vi "Teleop Climb Control.vi"(9 "D-Pad":T1, 10 "Button Cluster":T2, 11 "Axes":T3) -> ()   [LabVIEW 2017]
uses:
  Common Code/Gamepads/Axes Cluster.ctl
  Common Code/Gamepads/Button Cluster.ctl
  Common Code/Gamepads/D-Pad.ctl
  Common Code/Climb Command Cluster.ctl
  Common Code/Utilities/Change Detect.vi
  Common Code/Utilities/Change Detect Boolean.vi
  Robot Global Data.vi
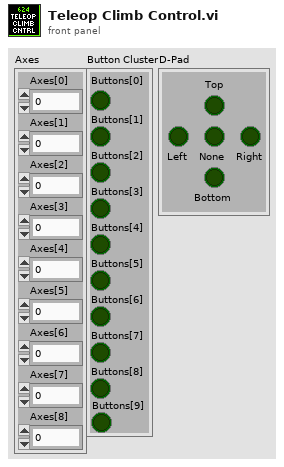
[diagram p1: front panel]
types:
  T1 = typedef "D-Pad.ctl" = cluster{"Top":bool, "Bottom":bool, "None":bool, "Right":bool, "Left":bool}
  T2 = typedef "Button Cluster.ctl" = cluster{"Buttons[0]":bool, "Buttons[1]":bool, "Buttons[2]":bool, "Buttons[3]":bool, "Buttons[4]":bool, "Buttons[5]":bool, "Buttons[6]":bool, "Buttons[7]":bool, "Buttons[8]":bool, "Buttons[9]":bool}
  T3 = typedef "Axes Cluster.ctl" = cluster{"Axes[0]":dbl, "Axes[1]":dbl, "Axes[2]":dbl, "Axes[3]":dbl, "Axes[4]":dbl, "Axes[5]":dbl, "Axes[6]":dbl, "Axes[7]":dbl, "Axes[8]":dbl}
  T4 = typedef "Climb Command Cluster.ctl" = cluster{"Climb":bool, "Button Pressed":bool}
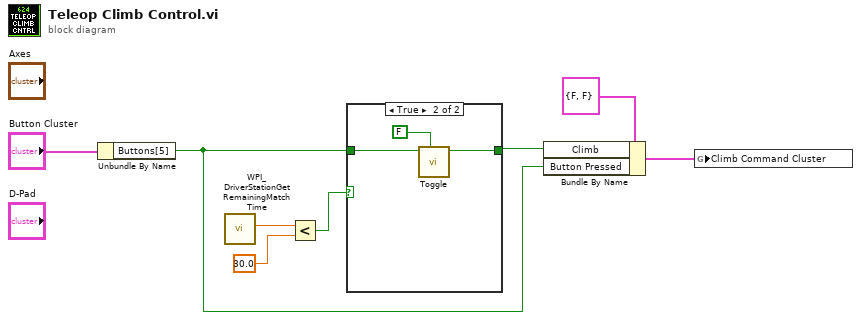
[diagram p0: block diagram]
diagram:
  n1 = Unbundle By Name("Button Cluster") -> ("Buttons[5]"=w2:bool)
  n2 = call <vilib>:"WPI_DriverStationGetRemainingMatchTime.vi"() -> ("Match Time(s)"=w1:sgl)  [unwired: 10 in, 1 out]
  n3 = Less?(x=w1, y=sgl 30.0) -> (x < y?=w3:bool)
  n4 = case shown="True" w3 {
    tunnel: [_ w9] -> w4
    tunnel: w2 -> [_ w10]
    frame False {
    }
    frame True {
      n5 = call "Toggle.vi"("Initial Value"=FALSE, "In"=w10) -> ("Toggled"=w9:bool)  [unwired: 9 in]
    }
  }
  n6 = Bundle By Name(cluster=T4 {"Climb"=FALSE, "Button Pressed"=FALSE} ("Climb Command Cluster"), "Climb"=w4, "Button Pressed"=w2) -> (w7:T4)
  n7 = global write "Robot Global Data.vi" "Climb Command Cluster"(w7) -> ()
